vi "Solve_Airstate.vi"() -> ()   [LabVIEW 2020]
uses:
  Utilities/Air Flow State.ctl
  Utilities/Air Constants.vi
panel:
  in  "Wet Bulb Temp [DegF]":dbl
  in  "Dry Bulb Temp [DegF]":dbl
  out "Complete Air Flow State":T1={"Flow Rate [CFM]"=0.0, "Pressure [psia]"=0.0, "Dry Bulb Temp [DegF]"=-460.0, "Wet Bulb Temp [DegF]"=-460.0, "Relative Humidity [%]"=-460.0, "Humidity Ratio [lbmv/lbma]"=-460.0, "Grains [Gr/lbma]"=-460.0, "Specific Volume [ft^3/lbma]"=-460.0, "Enthalpy [BTU/lbm]"=-460.0, "Dew Point [DegF]"=-460.0}
  in  "Elevation [ft]":dbl
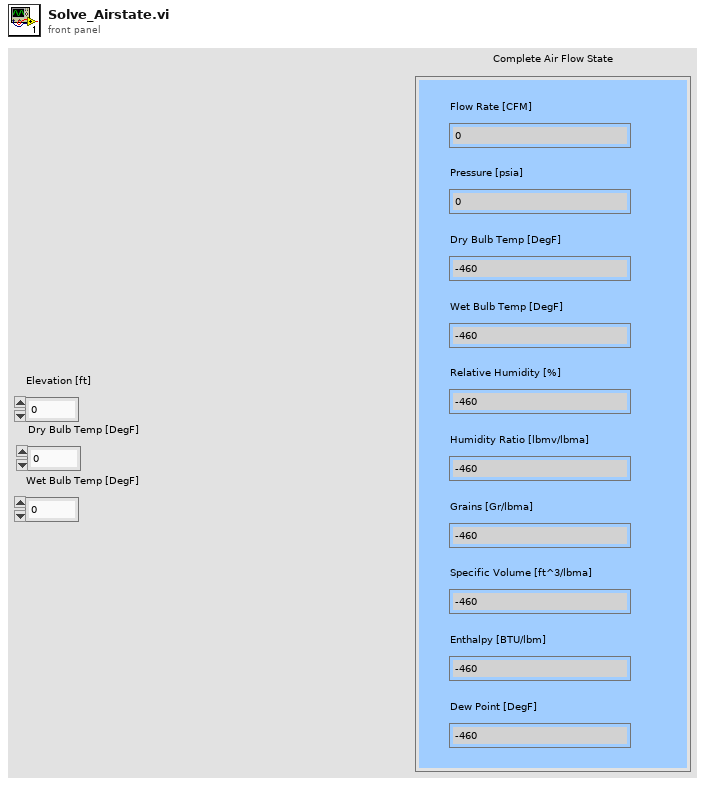
[diagram p1: front panel]
types:
  T1 = typedef "Air Flow State.ctl" = cluster{"Flow Rate [CFM]":dbl, "Pressure [psia]":dbl, "Dry Bulb Temp [DegF]":dbl, "Wet Bulb Temp [DegF]":dbl, "Relative Humidity [%]":dbl, "Humidity Ratio [lbmv/lbma]":dbl, "Grains [Gr/lbma]":dbl, "Specific Volume [ft^3/lbma]":dbl, "Enthalpy [BTU/lbm]":dbl, "Dew Point [DegF]":dbl}
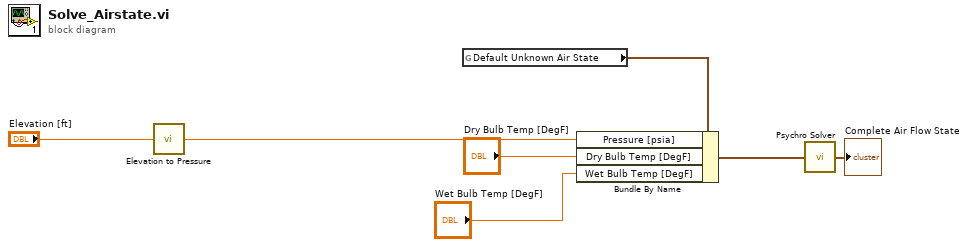
[diagram p0: block diagram]
diagram:
  n1 = call "Elevation to Pressure.vi"("Elevation [ft]"="Elevation [ft]") -> ("Pressure [psia]"=w5:dbl)
  n2 = global read "Air Constants.vi" "Default Unknown Air State"() -> (w6:T1)
  n3 = Bundle By Name(cluster=w6, "Pressure [psia]"=w5, "Dry Bulb Temp [DegF]"="Dry Bulb Temp [DegF]", "Wet Bulb Temp [DegF]"="Wet Bulb Temp [DegF]") -> (w7:T1)
  n4 = call "Psychro Solver.vi"("Incomplete Air Flow State"=w7) -> ("Complete Air Flow State"=→"Complete Air Flow State":T1)  [unwired: 14 in]
